vi "Run Time Program.vi"(8 "error in (no error)":errorcluster, 10 "SW":u16(ring) items=["A-B", "B-A", "A-C", "C-A", "B-C", "C-A"], 11 "VISA resource name":refnum<visa-resource-name>) -> (0 "error out":errorcluster, 3 "VISA resource name out":refnum<visa-resource-name>)   [LabVIEW 2021, in "BK Precision 169XB.lvlib"]
doc: "Configures over current protection (OCP). Specify the output current limit value and the behavior of the power supply when the output current is greater than or equal to that value."
uses:
  BK Precision 169XB.lvlib
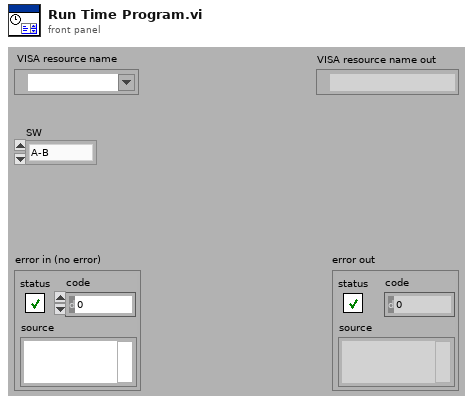
[diagram p1: front panel]
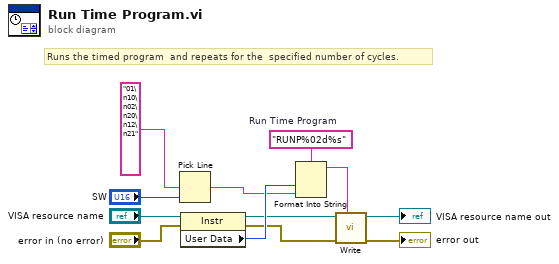
[diagram p0: block diagram]
diagram:
  w8 = "RUNP%02d%s"  # Run Time Program
  # "Runs the timed program  and repeats for the  specified number of cycles."
  n1 = Pick Line(multi-line string="01\n10\n02\n20\n12\n21", line index="SW") -> (output string=w2:string)  [unwired: 1 in]
  n2 = property class="Instr"(reference="VISA resource name", error in="error in (no error)") -> (reference out=w5:refnum<visa-resource-name>, error out=w4:errorcluster, "User Data"=w7:u32)
  n3 = Format Into String(format string=w8, w7, w2) -> (resulting string=w1:string)  [unwired: 2 in, 1 out]
  n4 = call "Write.vi"("Input String"=w1, "error in (no error)"=w4, "VISA resource name"=w5) -> ("error out"=→"error out":errorcluster, "VISA resource name out"=→"VISA resource name out":refnum<visa-resource-name>)  [unwired: 6 in, 1 out]
